vi "III_V_layer_v20.vi"(2 "Debug Mode":bool, 3 "Elapsed Time(s)":dbl, 4 "State":enum16{"Edit", "Start", "Run", "End", "Idle"}(ring), 5 "Argument List In":string[](array[string])) -> (0 "Status Out":string, 1 "Argument List Out":string[](array[string]))   [LabVIEW 2011]
uses:
  high_level_proc/Al_bubbler.ctl
  high_level_proc/In_bubbler.ctl
  high_level_proc/P_gas.ctl
  high_level_proc/As_gas.ctl
  high_level_proc/P_bubbler.ctl
  high_level_proc/bubblerDilution.ctl
panel:
  out "Zn bubbler Copy":T1={"Active"=FALSE, "main"={"Flow"=0.0, "Run"=FALSE, "Prep Ga"=FALSE, "Dilution"=FALSE, "Calculated"=0, "MFC2 flow"=10.0, "MFC3 flow"=100.0, "MFC1 flow"=0.0}} {"main"."MFC1 flow" format="%.4f"; "main"."MFC3 flow" format="%.1f"; "main"."MFC2 flow" format="%.2f"; "main"."Calculated" items=["Flow", "MFC1", "MFC2", "MFC3"]; "main"."Flow" format="%.2f"}
  in  "Zn bubbler":T1={"Active"=FALSE, "main"={"Flow"=0.0, "Run"=FALSE, "Prep Ga"=FALSE, "Dilution"=FALSE, "Calculated"=0, "MFC2 flow"=10.0, "MFC3 flow"=100.0, "MFC1 flow"=0.0}} {"main"."MFC1 flow" format="%.4f"; "main"."MFC3 flow" format="%.1f"; "main"."MFC2 flow" format="%.2f"; "main"."Calculated" items=["Flow", "MFC1", "MFC2", "MFC3"]; "main"."Flow" format="%.2f"}
  out "Se bubbler Copy":T1={"Active"=FALSE, "main"={"Flow"=0.0, "Run"=FALSE, "Prep Ga"=FALSE, "Dilution"=FALSE, "Calculated"=1, "MFC2 flow"=10.0, "MFC3 flow"=100.0, "MFC1 flow"=0.0}} {"main"."MFC1 flow" format="%.4f"; "main"."MFC3 flow" format="%.1f"; "main"."MFC2 flow" format="%.2f"; "main"."Calculated" items=["Ga flow", "MFC1", "MFC2", "MFC3"]; "main"."Flow" format="%.2f"}
  in  "Se bubbler":T1={"Active"=FALSE, "main"={"Flow"=0.0, "Run"=FALSE, "Prep Ga"=FALSE, "Dilution"=FALSE, "Calculated"=0, "MFC2 flow"=10.0, "MFC3 flow"=100.0, "MFC1 flow"=0.0}} {"main"."MFC1 flow" format="%.4f"; "main"."MFC3 flow" format="%.1f"; "main"."MFC2 flow" format="%.2f"; "main"."Calculated" items=["Flow", "MFC1", "MFC2", "MFC3"]; "main"."Flow" format="%.2f"}
  out "P bubbler Copy":T2 {"P bubbler main"."Flow" format="%.2f"}
  in  "P bubbler":T3 {"P bubbler main"."Flow" format="%.2f"}
  out "As gas Copy":T4 {"As gas main"."Flow" format="%.2f"}
  in  "As gas":T5 {"As gas main"."Flow" format="%.2f"}
  out "P gas Copy":T6 {"P gas main"."Flow" format="%.2f"}
  in  "P gas":T7 {"P gas main"."Flow" format="%.2f"}
  out "In bubbler Copy":T8 {"In main"."Flow" format="%.2f"}
  in  "In bubbler":T9 {"In main"."Flow" format="%.2f"}
  out "Ga bubbler Copy":T10={"Ga bubbler Active"=FALSE, "Ga main"={"Flow"=0.0, "Ga Run"=FALSE, "Prep Ga"=FALSE, "Dilution"=FALSE, "Ga Calculated"=1, "MFC2 flow"=10.0, "MFC3 flow"=100.0, "MFC1 flow"=0.0}} {"Ga main"."MFC1 flow" format="%.4f"; "Ga main"."MFC3 flow" format="%.1f"; "Ga main"."MFC2 flow" format="%.2f"; "Ga main"."Ga Calculated" items=["Ga flow", "MFC1", "MFC2", "MFC3"]; "Ga main"."Flow" format="%.2f"}
  in  "Ga bubbler":T1={"Active"=FALSE, "main"={"Flow"=0.0, "Run"=FALSE, "Prep Ga"=FALSE, "Dilution"=FALSE, "Calculated"=0, "MFC2 flow"=10.0, "MFC3 flow"=100.0, "MFC1 flow"=0.0}} {"main"."MFC1 flow" format="%.4f"; "main"."MFC3 flow" format="%.1f"; "main"."MFC2 flow" format="%.2f"; "main"."Calculated" items=["Flow", "MFC1", "MFC2", "MFC3"]; "main"."Flow" format="%.2f"}
  out "Al bubbler Copy":T11 {"Al main"."Al Flow" format="%.2f"}
  in  "Al bubbler":T12 {"Al main"."Al Flow" format="%.2f"}
  out "prep_done":bool
  out "run started":bool
  out "first":bool=TRUE
  out "total time":dbl
  out "is OK?":bool
  in  "prep_time":dbl
  in  "Cancel":bool
  in  "OK":bool
  out "tTotal(s) 2":dbl
  # "s"
  # "Add pre-run time to run time in editor."
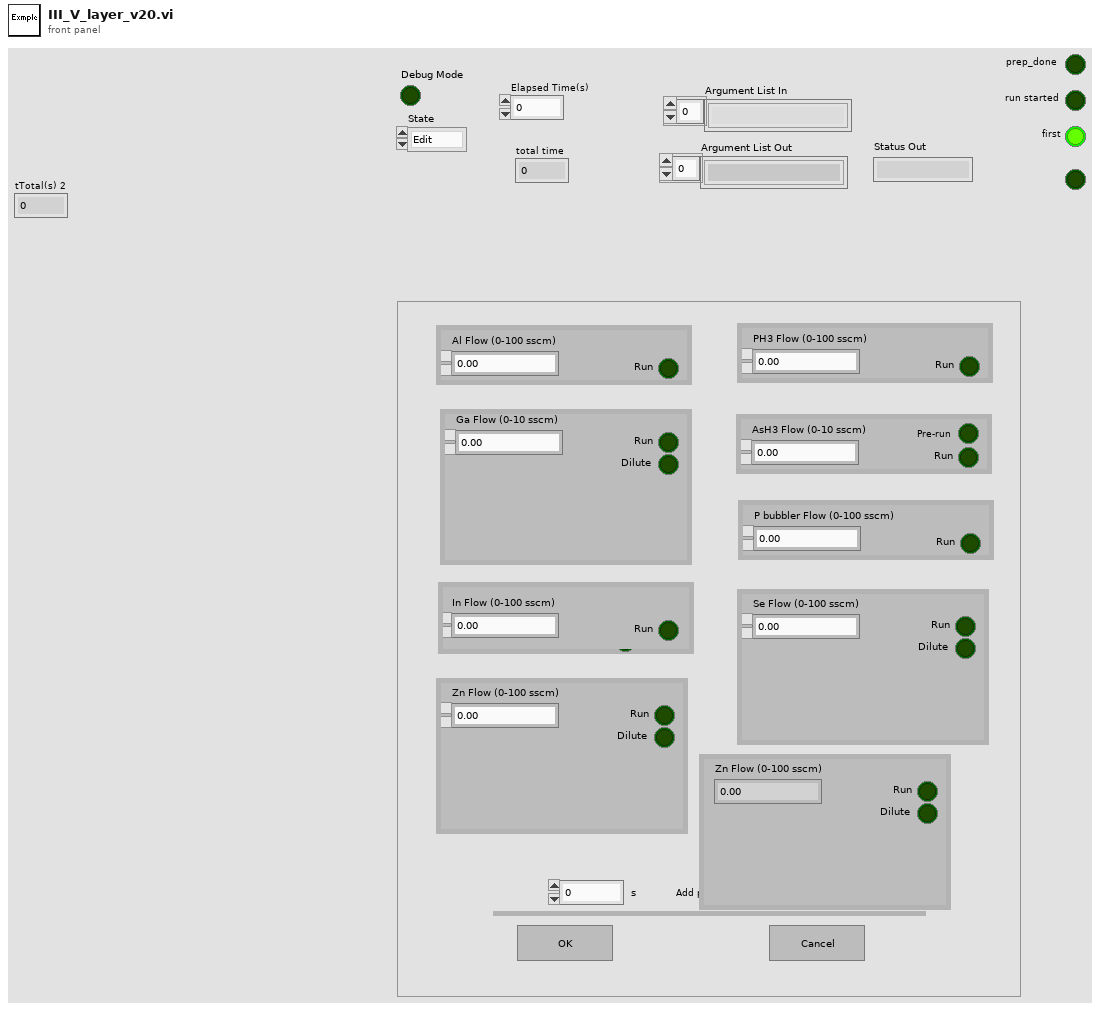
[diagram p1: front panel]
types:
  T1 = typedef "bubblerDilution.ctl" = cluster{"Active":bool, "main":cluster{"Flow":dbl, "Run":bool, "Prep Ga":bool, "Dilution":bool, "Calculated":u16, "MFC2 flow":dbl, "MFC3 flow":dbl, "MFC1 flow":dbl}}
  T2 = cluster{"P bubbler Active":bool, "P bubbler main":cluster{"Flow":dbl, "P bubbler Run":bool, "P bubbler Prep":bool}}
  T3 = typedef "P_bubbler.ctl" = cluster{"P bubbler Active":bool, "P bubbler main":cluster{"Flow":dbl, "P bubbler Run":bool, "P bubbler Prep":bool}}
  T4 = cluster{"As gas Active":bool, "As gas main":cluster{"Flow":dbl, "AsH3 Run":bool, "AsH3 Prep":bool}}
  T5 = typedef "As_gas.ctl" = cluster{"As gas Active":bool, "As gas main":cluster{"Flow":dbl, "AsH3 Run":bool, "AsH3 Prep":bool}}
  T6 = cluster{"P gas Active":bool, "P gas main":cluster{"Flow":dbl, "PH3 Run":bool, "PH3 Prep":bool}}
  T7 = typedef "P_gas.ctl" = cluster{"P gas Active":bool, "P gas main":cluster{"Flow":dbl, "PH3 Run":bool, "PH3 Prep":bool}}
  T8 = cluster{"In main":cluster{"Flow":dbl, "In Run":bool, "Prep In":bool}, "In bubbler Active":bool}
  T9 = typedef "In_bubbler.ctl" = cluster{"In main":cluster{"Flow":dbl, "In Run":bool, "Prep In":bool}, "In bubbler Active":bool}
  T10 = cluster{"Ga bubbler Active":bool, "Ga main":cluster{"Flow":dbl, "Ga Run":bool, "Prep Ga":bool, "Dilution":bool, "Ga Calculated":u16, "MFC2 flow":dbl, "MFC3 flow":dbl, "MFC1 flow":dbl}}
  T11 = cluster{"Al Active":bool, "Al main":cluster{"Al Flow":dbl, "Al Run":bool, "Prep Al":bool}}
  T12 = typedef "Al_bubbler.ctl" = cluster{"Al Active":bool, "Al main":cluster{"Al Flow":dbl, "Al Run":bool, "Prep Al":bool}}
  T13 = enum16{"Discrete", "Continuous", "Instantaneous", "Finite"}
  T14 = enum32{"Invalid", "Default", "Floating", "Floating/Auto-Hide", "Modal"}
  T15 = enum8{"Enabled", "Disabled", "Disabled and Grayed Out"}
  T16 = cluster{"Active":bool, "main":cluster{"Flow":dbl, "Run":bool, "Prep Ga":bool, "Dilution":bool, "Calculated":u16, "MFC2 flow":dbl, "MFC3 flow":dbl, "MFC1 flow":dbl}}
  T17 = cluster{"Al Flow":dbl, "Al Run":bool, "Prep Al":bool}
  T18 = cluster{"Flow":dbl, "Run":bool, "Prep Ga":bool, "Dilution":bool, "Calculated":u16, "MFC2 flow":dbl, "MFC3 flow":dbl, "MFC1 flow":dbl}
  T19 = cluster{"Flow":dbl, "In Run":bool, "Prep In":bool}
  T20 = cluster{"Flow":dbl, "PH3 Run":bool, "PH3 Prep":bool}
  T21 = cluster{"Flow":dbl, "AsH3 Run":bool, "AsH3 Prep":bool}
  T22 = cluster{"Flow":dbl, "P bubbler Run":bool, "P bubbler Prep":bool}
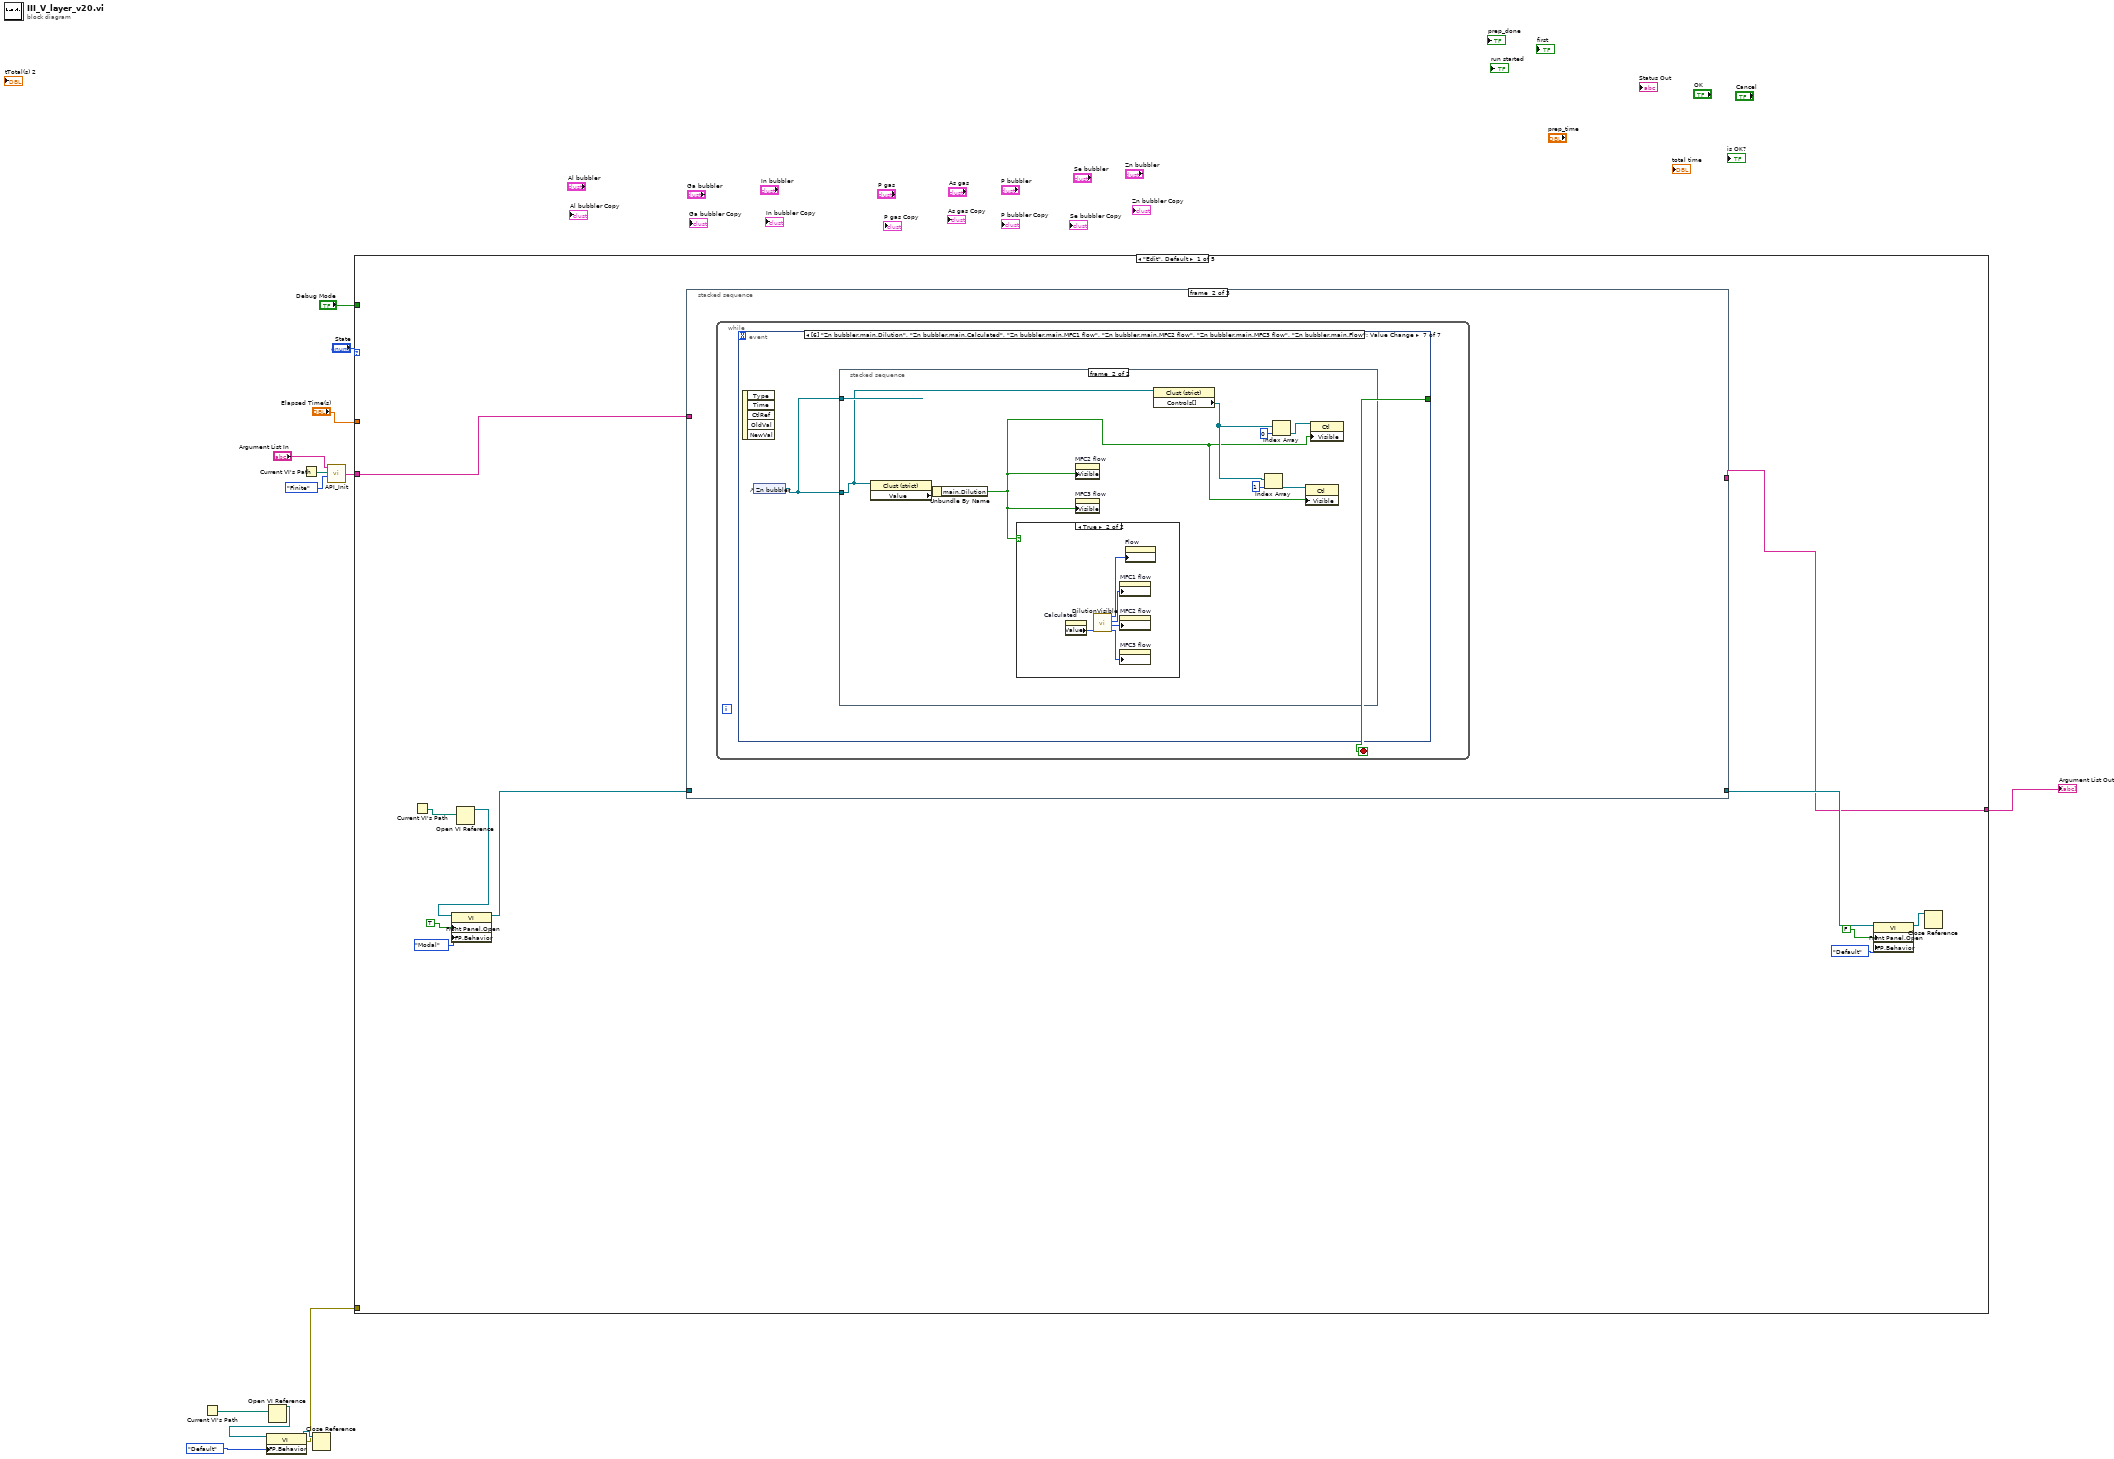
[diagram p0: block diagram]
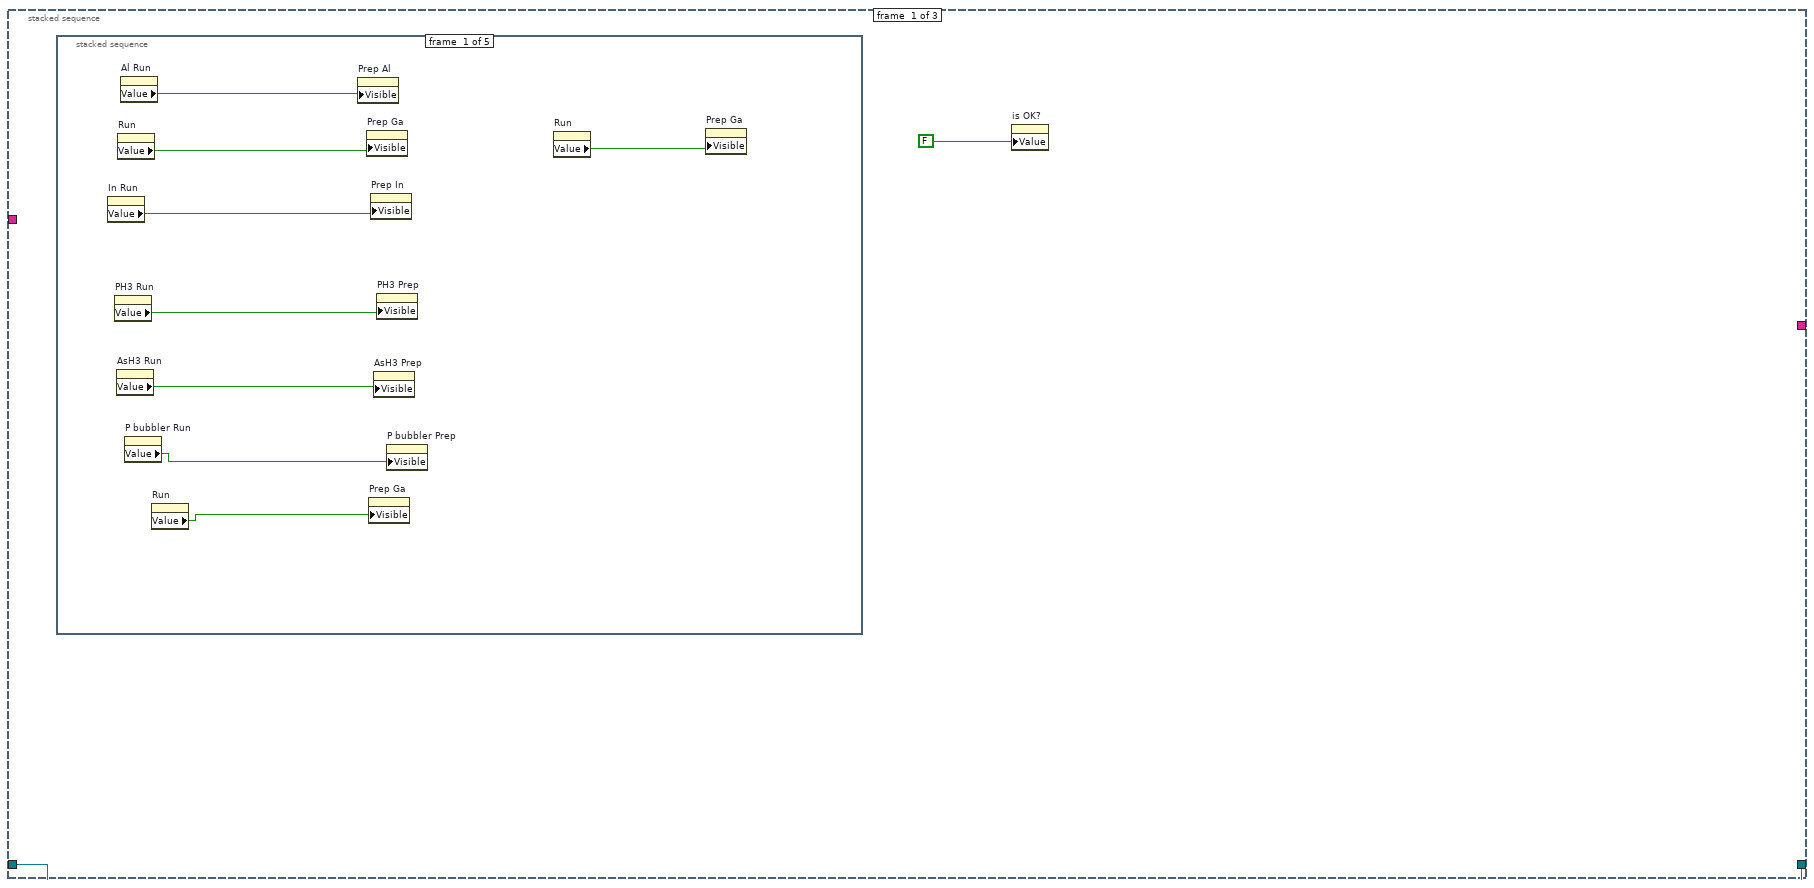
[diagram p2: hidden frame]
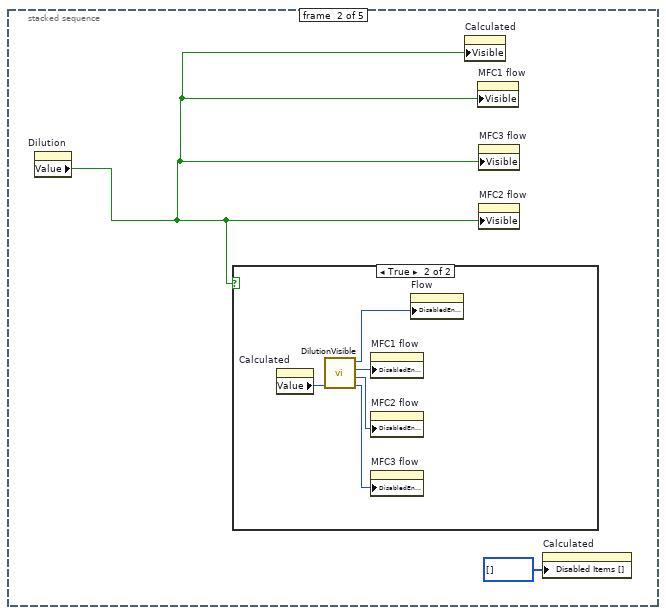
[diagram p3: hidden frame]
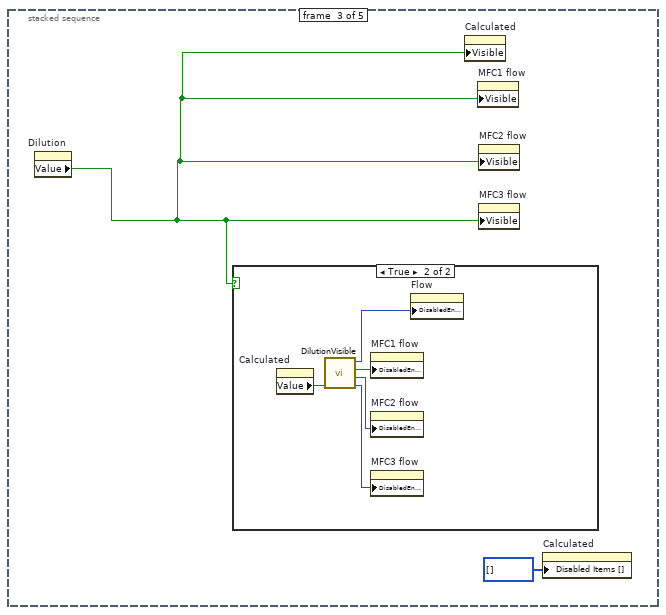
[diagram p5: hidden frame]
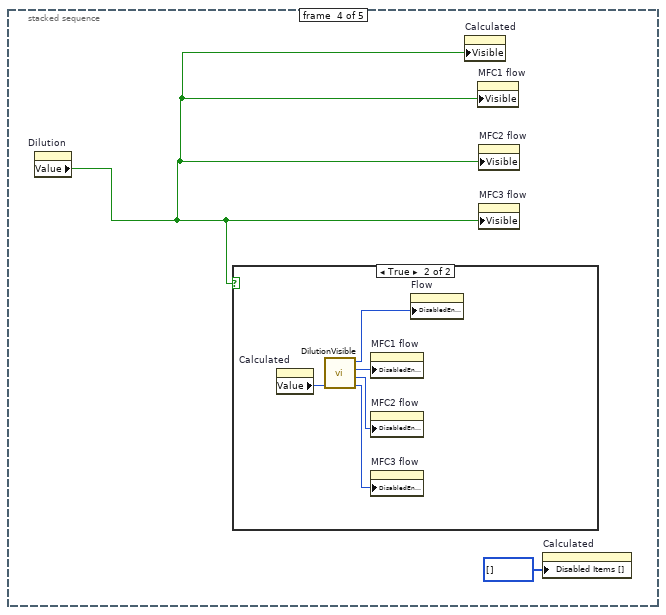
[diagram p7: hidden frame]
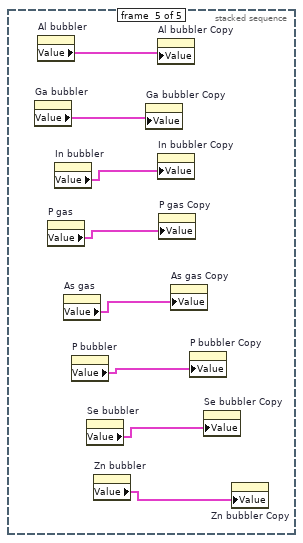
[diagram p9: hidden frame]
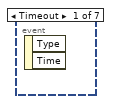
[diagram p10: hidden frame]
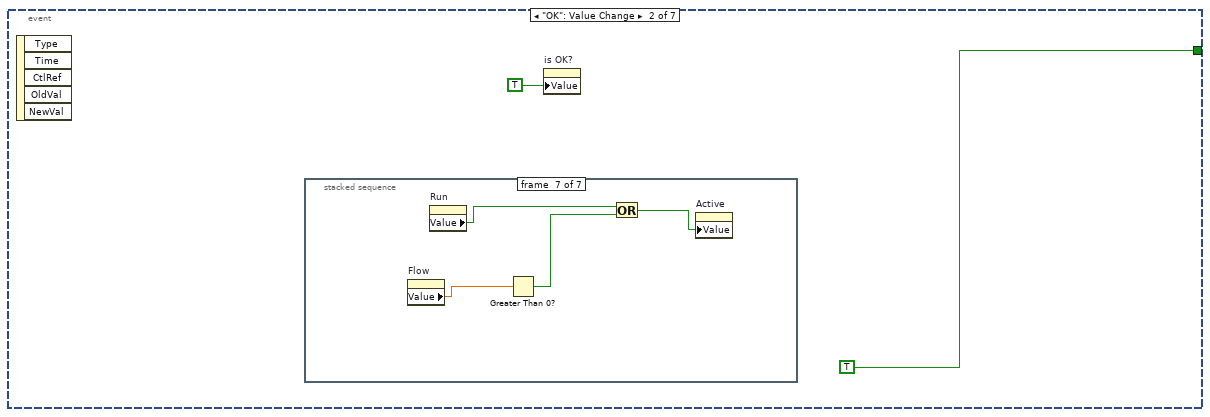
[diagram p11: hidden frame]
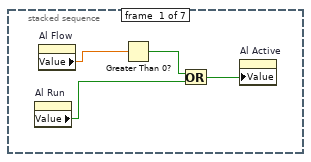
[diagram p12: hidden frame]
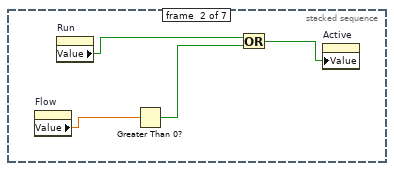
[diagram p13: hidden frame]
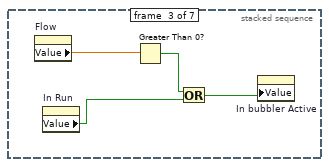
[diagram p14: hidden frame]
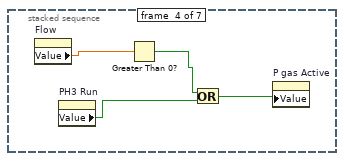
[diagram p15: hidden frame]
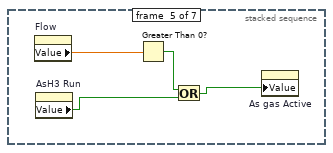
[diagram p16: hidden frame]
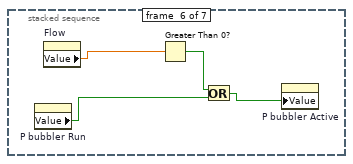
[diagram p17: hidden frame]
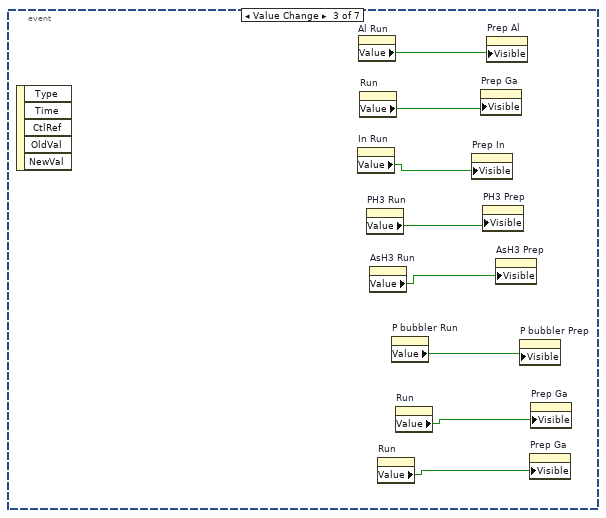
[diagram p18: hidden frame]
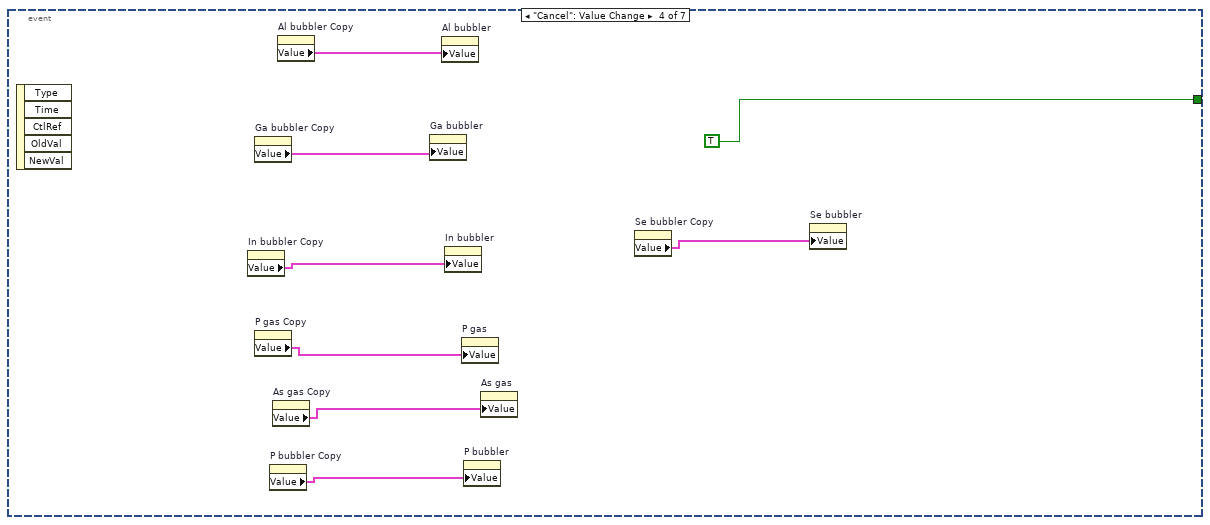
[diagram p19: hidden frame]
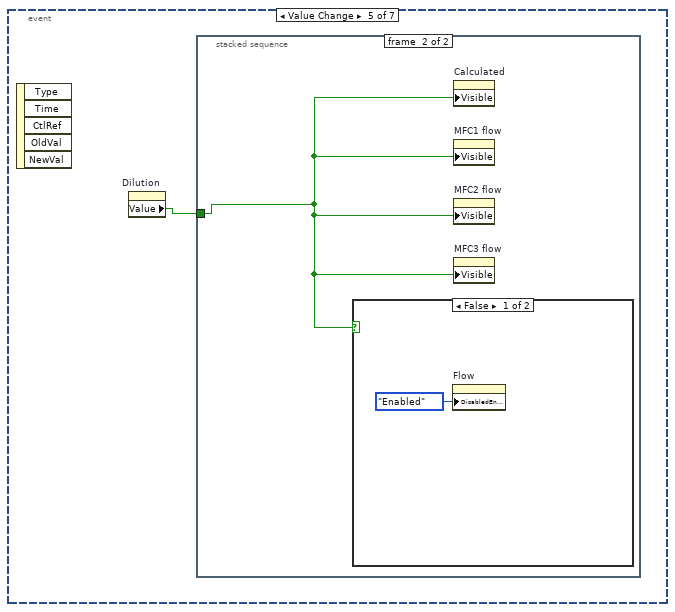
[diagram p20: hidden frame]
diagram:
  n1 = Current VI's Path() -> (path=w9:path)
  n2 = Open VI Reference(vi path=w9) -> (vi reference=w8:refnum<vi>)  [unwired: 1 in, 5 out]
  n3 = property class="VI"(reference=w8, "FP.Behavior"=T14."Default" ("Front Panel Window:Behavior")) -> (reference out=w6:refnum<vi>, error out=w5:errorcluster)  [unwired: 1 in]
  n4 = Current VI's Path() -> (path=w4:path)
  n5 = Close Reference(reference=w6) -> ()  [unwired: 1 in, 1 out]
  n6 = call "API_Init.vi"("API Mode"=T13."Finite", "VI Path"=w4, "Argument List In"="Argument List In") -> ("Argument List Out"=w1:string[])  [unwired: 1 in]
  n7 = case shown="\"Edit\", Default" "State" {
    tunnel: "Debug Mode" -> [_ w191 w208 _ _]
    tunnel: "Elapsed Time(s)" -> [_ _ w209 _ _]
    tunnel: w1 -> [w15 w195 w207 w318 w319]
    tunnel: [w14 w194 w206 w318 w319] -> w10
    tunnel: w5 -> [_ _ _ _ _]
    frame "Edit", Default {
      n8 = Current VI's Path() -> (path=w20:path)
      n9 = Open VI Reference(vi path=w20) -> (vi reference=w19:refnum<vi>)  [unwired: 1 in, 5 out]
      n10 = property class="VI"(reference=w19, "Front Panel.Open"=TRUE ("Front Panel Window:Open"), "FP.Behavior"=T14."Modal" ("Front Panel Window:Behavior")) -> (reference out=w18:refnum<vi>)  [unwired: 1 in, 1 out]
      n11 = stacked-sequence {
        tunnel: w15 -> [_ _ w186]
        tunnel: w18 -> [w26 _ _]
        tunnel: [w26 _ _] -> w22
        tunnel: [_ _ w187] -> w14
        frame #0 {
          n12 = stacked-sequence {
            frame #0 {
              n13 = property on="In Run" class="Bool (strict)"() -> ("Value"=w33:bool)  [unwired: 2 in, 2 out]
              n14 = property on="PH3 Run" class="Bool (strict)"() -> ("Value"=w31:bool)  [unwired: 2 in, 2 out]
              n15 = property on="AsH3 Run" class="Bool (strict)"() -> ("Value"=w30:bool)  [unwired: 2 in, 2 out]
              n16 = property on="Run" class="Bool (strict)"() -> ("Value"=w32:bool)  [unwired: 2 in, 2 out]
              n17 = property on="Al Run" class="Bool (strict)"() -> ("Value"=w34:bool)  [unwired: 2 in, 2 out]
              n18 = property on="P bubbler Run" class="Bool (strict)"() -> ("Value"=w29:bool)  [unwired: 2 in, 2 out]
              n19 = property on="Run" class="Bool (strict)"() -> ("Value"=w28:bool)  [unwired: 2 in, 2 out]
              n20 = property on="Prep Al" class="Bool (strict)"("Visible"=w34) -> ()  [unwired: 2 in, 2 out]
              n21 = property on="Prep Ga" class="Bool (strict)"("Visible"=w32) -> ()  [unwired: 2 in, 2 out]
              n22 = property on="Prep Ga" class="Bool (strict)"("Visible"=w28) -> ()  [unwired: 2 in, 2 out]
              n23 = property on="Prep In" class="Bool (strict)"("Visible"=w33) -> ()  [unwired: 2 in, 2 out]
              n24 = property on="AsH3 Prep" class="Bool (strict)"("Visible"=w30) -> ()  [unwired: 2 in, 2 out]
              n25 = property on="PH3 Prep" class="Bool (strict)"("Visible"=w31) -> ()  [unwired: 2 in, 2 out]
              n26 = property on="P bubbler Prep" class="Bool (strict)"("Visible"=w29) -> ()  [unwired: 2 in, 2 out]
              n27 = property on="Run" class="Bool (strict)"() -> ("Value"=w27:bool)  [unwired: 2 in, 2 out]
              n28 = property on="Prep Ga" class="Bool (strict)"("Visible"=w27) -> ()  [unwired: 2 in, 2 out]
            }
            frame #1 {
              n29 = property on="Dilution" class="Bool (strict)"() -> ("Value"=w36:bool)  [unwired: 2 in, 2 out]
              n30 = case shown="True" w36 {
                frame False {
                }
                frame True {
                  n31 = property on="Calculated" class="Ring (strict)"() -> ("Value"=w37:u16)  [unwired: 2 in, 2 out]
                  n32 = call "DilutionVisible.vi"("calculated"=w37) -> ("MFC3"=w40:u16, "MFC2"=w39:u16, "MFC1"=w38:u16, "flow"=w41:u16)  [unwired: 3 in]
                  n33 = property on="MFC1 flow" class="DigNum (strict)"("DisabledEnum"=w38) -> ()  [unwired: 2 in, 2 out]
                  n34 = property on="MFC2 flow" class="DigNum (strict)"("DisabledEnum"=w39) -> ()  [unwired: 2 in, 2 out]
                  n35 = property on="MFC3 flow" class="DigNum (strict)"("DisabledEnum"=w40) -> ()  [unwired: 2 in, 2 out]
                  n36 = property on="Flow" class="DigNum (strict)"("DisabledEnum"=w41) -> ()  [unwired: 2 in, 2 out]
                }
              }
              n37 = property on="Calculated" class="Ring (strict)"("Visible"=w36) -> ()  [unwired: 2 in, 2 out]
              n38 = property on="MFC1 flow" class="DigNum (strict)"("Visible"=w36) -> ()  [unwired: 2 in, 2 out]
              n39 = property on="MFC3 flow" class="DigNum (strict)"("Visible"=w36) -> ()  [unwired: 2 in, 2 out]
              n40 = property on="MFC2 flow" class="DigNum (strict)"("Visible"=w36) -> ()  [unwired: 2 in, 2 out]
              n41 = property on="Calculated" class="Ring (strict)"("Disabled Items []"=i32[] []) -> ()  [unwired: 2 in, 2 out]
            }
            frame #2 {
              n42 = property on="Dilution" class="Bool (strict)"() -> ("Value"=w43:bool)  [unwired: 2 in, 2 out]
              n43 = case shown="True" w43 {
                frame False {
                }
                frame True {
                  n44 = property on="Calculated" class="Ring (strict)"() -> ("Value"=w44:u16)  [unwired: 2 in, 2 out]
                  n45 = call "DilutionVisible.vi"("calculated"=w44) -> ("MFC3"=w47:u16, "MFC2"=w46:u16, "MFC1"=w45:u16, "flow"=w48:u16)  [unwired: 3 in]
                  n46 = property on="MFC1 flow" class="DigNum (strict)"("DisabledEnum"=w45) -> ()  [unwired: 2 in, 2 out]
                  n47 = property on="MFC2 flow" class="DigNum (strict)"("DisabledEnum"=w46) -> ()  [unwired: 2 in, 2 out]
                  n48 = property on="MFC3 flow" class="DigNum (strict)"("DisabledEnum"=w47) -> ()  [unwired: 2 in, 2 out]
                  n49 = property on="Flow" class="DigNum (strict)"("DisabledEnum"=w48) -> ()  [unwired: 2 in, 2 out]
                }
              }
              n50 = property on="Calculated" class="Ring (strict)"("Visible"=w43) -> ()  [unwired: 2 in, 2 out]
              n51 = property on="MFC1 flow" class="DigNum (strict)"("Visible"=w43) -> ()  [unwired: 2 in, 2 out]
              n52 = property on="MFC2 flow" class="DigNum (strict)"("Visible"=w43) -> ()  [unwired: 2 in, 2 out]
              n53 = property on="MFC3 flow" class="DigNum (strict)"("Visible"=w43) -> ()  [unwired: 2 in, 2 out]
              n54 = property on="Calculated" class="Ring (strict)"("Disabled Items []"=i32[] []) -> ()  [unwired: 2 in, 2 out]
            }
            frame #3 {
              n55 = property on="Dilution" class="Bool (strict)"() -> ("Value"=w50:bool)  [unwired: 2 in, 2 out]
              n56 = case shown="True" w50 {
                frame False {
                }
                frame True {
                  n57 = property on="Calculated" class="Ring (strict)"() -> ("Value"=w51:u16)  [unwired: 2 in, 2 out]
                  n58 = call "DilutionVisible.vi"("calculated"=w51) -> ("MFC3"=w54:u16, "MFC2"=w53:u16, "MFC1"=w52:u16, "flow"=w55:u16)  [unwired: 3 in]
                  n59 = property on="MFC1 flow" class="DigNum (strict)"("DisabledEnum"=w52) -> ()  [unwired: 2 in, 2 out]
                  n60 = property on="MFC2 flow" class="DigNum (strict)"("DisabledEnum"=w53) -> ()  [unwired: 2 in, 2 out]
                  n61 = property on="MFC3 flow" class="DigNum (strict)"("DisabledEnum"=w54) -> ()  [unwired: 2 in, 2 out]
                  n62 = property on="Flow" class="DigNum (strict)"("DisabledEnum"=w55) -> ()  [unwired: 2 in, 2 out]
                }
              }
              n63 = property on="Calculated" class="Ring (strict)"("Visible"=w50) -> ()  [unwired: 2 in, 2 out]
              n64 = property on="MFC1 flow" class="DigNum (strict)"("Visible"=w50) -> ()  [unwired: 2 in, 2 out]
              n65 = property on="MFC2 flow" class="DigNum (strict)"("Visible"=w50) -> ()  [unwired: 2 in, 2 out]
              n66 = property on="MFC3 flow" class="DigNum (strict)"("Visible"=w50) -> ()  [unwired: 2 in, 2 out]
              n67 = property on="Calculated" class="Ring (strict)"("Disabled Items []"=i32[] []) -> ()  [unwired: 2 in, 2 out]
            }
            frame #4 {
              n68 = property on="Ga bubbler" class="Clust (strict)"() -> ("Value"=w62:T16)  [unwired: 2 in, 2 out]
              n69 = property on="Al bubbler" class="Clust (strict)"() -> ("Value"=w63:T11)  [unwired: 2 in, 2 out]
              n70 = property on="P gas" class="Clust (strict)"() -> ("Value"=w60:T6)  [unwired: 2 in, 2 out]
              n71 = property on="In bubbler" class="Clust (strict)"() -> ("Value"=w61:T8)  [unwired: 2 in, 2 out]
              n72 = property on="As gas" class="Clust (strict)"() -> ("Value"=w59:T4)  [unwired: 2 in, 2 out]
              n73 = property on="P bubbler" class="Clust (strict)"() -> ("Value"=w58:T2)  [unwired: 2 in, 2 out]
              n74 = property on="Se bubbler" class="Clust (strict)"() -> ("Value"=w57:T16)  [unwired: 2 in, 2 out]
              n75 = property on="Zn bubbler" class="Clust (strict)"() -> ("Value"=w56:T16)  [unwired: 2 in, 2 out]
              n76 = property on="Ga bubbler Copy" class="Clust (strict)"("Value"=w62) -> ()  [unwired: 2 in, 2 out]
              n77 = property on="Al bubbler Copy" class="Clust (strict)"("Value"=w63) -> ()  [unwired: 2 in, 2 out]
              n78 = property on="In bubbler Copy" class="Clust (strict)"("Value"=w61) -> ()  [unwired: 2 in, 2 out]
              n79 = property on="P gas Copy" class="Clust (strict)"("Value"=w60) -> ()  [unwired: 2 in, 2 out]
              n80 = property on="As gas Copy" class="Clust (strict)"("Value"=w59) -> ()  [unwired: 2 in, 2 out]
              n81 = property on="P bubbler Copy" class="Clust (strict)"("Value"=w58) -> ()  [unwired: 2 in, 2 out]
              n82 = property on="Se bubbler Copy" class="Clust (strict)"("Value"=w57) -> ()  [unwired: 2 in, 2 out]
              n83 = property on="Zn bubbler Copy" class="Clust (strict)"("Value"=w56) -> ()  [unwired: 2 in, 2 out]
            }
          }
          n84 = property on="is OK?" class="Bool (strict)"("Value"=FALSE ("is OK?")) -> ()  [unwired: 2 in, 2 out]
        }
        frame #1 {
          n85 = while {
            stop <- w64 stop-if-true
            n86 = event shown="[6] \"Zn bubbler.main.Dilution\", \"Zn bubbler.main.Calculated\", \"Zn bubbler.main.MFC1 flow\", \"Zn bubbler.main.MFC2 flow\", \"Zn bubbler.main.MFC3 flow\", \"Zn bubbler.main.Flow\": Value Change" {
              selector: _ -> [_ _ _ _ _ _ _]
              dyn-events: _ -> [_ _ _ _ _ _ _]
              timeout: _ -> [_ _ _ _ _ _ _]
              tunnel: [_ TRUE _ TRUE _ _ _] -> w64
              event Timeout {
                n87 = event-data() -> ()  [unwired: 1 in, 2 out]
              }
              event "OK": Value Change {
                n88 = event-data() -> ()  [unwired: 1 in, 5 out]
                n89 = stacked-sequence {
                  frame #0 {
                    n90 = property on="Al Run" class="Bool (strict)"() -> ("Value"=w68:bool)  [unwired: 2 in, 2 out]
                    n91 = property on="Al Flow" class="DigNum (strict)"() -> ("Value"=w69:dbl)  [unwired: 2 in, 2 out]
                    n92 = Greater Than 0?(x=w69) -> (x > 0?=w70:bool)
                    n93 = Or(x=w70, y=w68) -> (x .or. y?=w67:bool)
                    n94 = property on="Al Active" class="Bool (strict)"("Value"=w67) -> ()  [unwired: 2 in, 2 out]
                  }
                  frame #1 {
                    n95 = property on="Flow" class="DigNum (strict)"() -> ("Value"=w71:dbl)  [unwired: 2 in, 2 out]
                    n96 = property on="Run" class="Bool (strict)"() -> ("Value"=w72:bool)  [unwired: 2 in, 2 out]
                    n97 = Greater Than 0?(x=w71) -> (x > 0?=w74:bool)
                    n98 = Or(x=w72, y=w74) -> (x .or. y?=w73:bool)
                    n99 = property on="Active" class="Bool (strict)"("Value"=w73) -> ()  [unwired: 2 in, 2 out]
                  }
                  frame #2 {
                    n100 = property on="Flow" class="DigNum (strict)"() -> ("Value"=w77:dbl)  [unwired: 2 in, 2 out]
                    n101 = property on="In Run" class="Bool (strict)"() -> ("Value"=w76:bool)  [unwired: 2 in, 2 out]
                    n102 = Greater Than 0?(x=w77) -> (x > 0?=w78:bool)
                    n103 = Or(x=w78, y=w76) -> (x .or. y?=w75:bool)
                    n104 = property on="In bubbler Active" class="Bool (strict)"("Value"=w75) -> ()  [unwired: 2 in, 2 out]
                  }
                  frame #3 {
                    n105 = property on="Flow" class="DigNum (strict)"() -> ("Value"=w81:dbl)  [unwired: 2 in, 2 out]
                    n106 = property on="PH3 Run" class="Bool (strict)"() -> ("Value"=w80:bool)  [unwired: 2 in, 2 out]
                    n107 = Greater Than 0?(x=w81) -> (x > 0?=w82:bool)
                    n108 = Or(x=w82, y=w80) -> (x .or. y?=w79:bool)
                    n109 = property on="P gas Active" class="Bool (strict)"("Value"=w79) -> ()  [unwired: 2 in, 2 out]
                  }
                  frame #4 {
                    n110 = property on="Flow" class="DigNum (strict)"() -> ("Value"=w85:dbl)  [unwired: 2 in, 2 out]
                    n111 = property on="AsH3 Run" class="Bool (strict)"() -> ("Value"=w84:bool)  [unwired: 2 in, 2 out]
                    n112 = Greater Than 0?(x=w85) -> (x > 0?=w86:bool)
                    n113 = Or(x=w86, y=w84) -> (x .or. y?=w83:bool)
                    n114 = property on="As gas Active" class="Bool (strict)"("Value"=w83) -> ()  [unwired: 2 in, 2 out]
                  }
                  frame #5 {
                    n115 = property on="P bubbler Run" class="Bool (strict)"() -> ("Value"=w88:bool)  [unwired: 2 in, 2 out]
                    n116 = property on="Flow" class="DigNum (strict)"() -> ("Value"=w89:dbl)  [unwired: 2 in, 2 out]
                    n117 = Greater Than 0?(x=w89) -> (x > 0?=w90:bool)
                    n118 = Or(x=w90, y=w88) -> (x .or. y?=w87:bool)
                    n119 = property on="P bubbler Active" class="Bool (strict)"("Value"=w87) -> ()  [unwired: 2 in, 2 out]
                  }
                  frame #6 {
                    n120 = property on="Flow" class="DigNum (strict)"() -> ("Value"=w91:dbl)  [unwired: 2 in, 2 out]
                    n121 = property on="Run" class="Bool (strict)"() -> ("Value"=w92:bool)  [unwired: 2 in, 2 out]
                    n122 = Greater Than 0?(x=w91) -> (x > 0?=w94:bool)
                    n123 = Or(x=w92, y=w94) -> (x .or. y?=w93:bool)
                    n124 = property on="Active" class="Bool (strict)"("Value"=w93) -> ()  [unwired: 2 in, 2 out]
                  }
                }
                n125 = property on="is OK?" class="Bool (strict)"("Value"=TRUE ("is OK?")) -> ()  [unwired: 2 in, 2 out]
              }
              event Value Change {
                n126 = event-data() -> ()  [unwired: 1 in, 5 out]
                n127 = property on="In Run" class="Bool (strict)"() -> ("Value"=w99:bool)  [unwired: 2 in, 2 out]
                n128 = property on="Al Run" class="Bool (strict)"() -> ("Value"=w101:bool)  [unwired: 2 in, 2 out]
                n129 = property on="Run" class="Bool (strict)"() -> ("Value"=w100:bool)  [unwired: 2 in, 2 out]
                n130 = property on="PH3 Run" class="Bool (strict)"() -> ("Value"=w98:bool)  [unwired: 2 in, 2 out]
                n131 = property on="AsH3 Run" class="Bool (strict)"() -> ("Value"=w97:bool)  [unwired: 2 in, 2 out]
                n132 = property on="Run" class="Bool (strict)"() -> ("Value"=w95:bool)  [unwired: 2 in, 2 out]
                n133 = property on="P bubbler Run" class="Bool (strict)"() -> ("Value"=w102:bool)  [unwired: 2 in, 2 out]
                n134 = property on="Run" class="Bool (strict)"() -> ("Value"=w96:bool)  [unwired: 2 in, 2 out]
                n135 = property on="Prep In" class="Bool (strict)"("Visible"=w99) -> ()  [unwired: 2 in, 2 out]
                n136 = property on="Prep Ga" class="Bool (strict)"("Visible"=w100) -> ()  [unwired: 2 in, 2 out]
                n137 = property on="PH3 Prep" class="Bool (strict)"("Visible"=w98) -> ()  [unwired: 2 in, 2 out]
                n138 = property on="Prep Al" class="Bool (strict)"("Visible"=w101) -> ()  [unwired: 2 in, 2 out]
                n139 = property on="AsH3 Prep" class="Bool (strict)"("Visible"=w97) -> ()  [unwired: 2 in, 2 out]
                n140 = property on="P bubbler Prep" class="Bool (strict)"("Visible"=w102) -> ()  [unwired: 2 in, 2 out]
                n141 = property on="Prep Ga" class="Bool (strict)"("Visible"=w95) -> ()  [unwired: 2 in, 2 out]
                n142 = property on="Prep Ga" class="Bool (strict)"("Visible"=w96) -> ()  [unwired: 2 in, 2 out]
              }
              event "Cancel": Value Change {
                n143 = event-data() -> ()  [unwired: 1 in, 5 out]
                n144 = property on="In bubbler Copy" class="Clust (strict)"() -> ("Value"=w108:T8)  [unwired: 2 in, 2 out]
                n145 = property on="Ga bubbler Copy" class="Clust (strict)"() -> ("Value"=w107:T10)  [unwired: 2 in, 2 out]
                n146 = property on="P gas Copy" class="Clust (strict)"() -> ("Value"=w106:T6)  [unwired: 2 in, 2 out]
                n147 = property on="P bubbler Copy" class="Clust (strict)"() -> ("Value"=w104:T2)  [unwired: 2 in, 2 out]
                n148 = property on="As gas Copy" class="Clust (strict)"() -> ("Value"=w105:T4)  [unwired: 2 in, 2 out]
                n149 = property on="Al bubbler Copy" class="Clust (strict)"() -> ("Value"=w109:T11)  [unwired: 2 in, 2 out]
                n150 = property on="Ga bubbler" class="Clust (strict)"("Value"=w107) -> ()  [unwired: 2 in, 2 out]
                n151 = property on="Al bubbler" class="Clust (strict)"("Value"=w109) -> ()  [unwired: 2 in, 2 out]
                n152 = property on="In bubbler" class="Clust (strict)"("Value"=w108) -> ()  [unwired: 2 in, 2 out]
                n153 = property on="P gas" class="Clust (strict)"("Value"=w106) -> ()  [unwired: 2 in, 2 out]
                n154 = property on="P bubbler" class="Clust (strict)"("Value"=w104) -> ()  [unwired: 2 in, 2 out]
                n155 = property on="As gas" class="Clust (strict)"("Value"=w105) -> ()  [unwired: 2 in, 2 out]
                n156 = property on="Se bubbler Copy" class="Clust (strict)"() -> ("Value"=w103:T16)  [unwired: 2 in, 2 out]
                n157 = property on="Se bubbler" class="Clust (strict)"("Value"=w103) -> ()  [unwired: 2 in, 2 out]
              }
              event Value Change {
                n158 = event-data() -> ()  [unwired: 1 in, 5 out]
                n159 = property on="Dilution" class="Bool (strict)"() -> ("Value"=w111:bool)  [unwired: 2 in, 2 out]
                n160 = stacked-sequence {
                  tunnel: w111 -> [w112 w122]
                  frame #0 {
                    n161 = case shown="True" w112 {
                      frame False {
                      }
                      frame True {
                        n162 = property on="Flow" class="DigNum (strict)"() -> ("Value"=w120:dbl)  [unwired: 2 in, 2 out]
                        n163 = property on="Calculated" class="Ring (strict)"() -> ("Value"=w121:u16)  [unwired: 2 in, 2 out]
                        n164 = property on="MFC1 flow" class="DigNum (strict)"() -> ("Value"=w119:dbl)  [unwired: 2 in, 2 out]
                        n165 = property on="MFC2 flow" class="DigNum (strict)"() -> ("Value"=w118:dbl)  [unwired: 2 in, 2 out]
                        n166 = property on="MFC3 flow" class="DigNum (strict)"() -> ("Value"=w117:dbl)  [unwired: 2 in, 2 out]
                        n167 = call "dilutionCalc.vi"("Calculated"=w121, "MFC3"=w117, "MFC2"=w118, "MFC1"=w119, "flow"=w120) -> ("MFC3 out"=w113:dbl, "MFC2 out"=w114:dbl, "MFC1 out"=w115:dbl, "flow out"=w116:dbl)  [unwired: 1 in]
                        n168 = property on="MFC1 flow" class="DigNum (strict)"("Value"=w115) -> ()  [unwired: 2 in, 2 out]
                        n169 = property on="Flow" class="DigNum (strict)"("Value"=w116) -> ()  [unwired: 2 in, 2 out]
                        n170 = property on="MFC3 flow" class="DigNum (strict)"("Value"=w113) -> ()  [unwired: 2 in, 2 out]
                        n171 = property on="MFC2 flow" class="DigNum (strict)"("Value"=w114) -> ()  [unwired: 2 in, 2 out]
                      }
                    }
                  }
                  frame #1 {
                    n172 = case shown="False" w122 {
                      frame False {
                        n173 = property on="Flow" class="DigNum (strict)"("DisabledEnum"=T15."Enabled" ("Disabled")) -> ()  [unwired: 2 in, 2 out]
                      }
                      frame True {
                        n174 = property on="Calculated" class="Ring (strict)"() -> ("Value"=w124:u16)  [unwired: 2 in, 2 out]
                        n175 = call "DilutionVisible.vi"("calculated"=w124) -> ("MFC3"=w128:u16, "MFC2"=w127:u16, "MFC1"=w126:u16, "flow"=w125:u16)  [unwired: 3 in]
                        n176 = property on="MFC1 flow" class="DigNum (strict)"("DisabledEnum"=w126) -> ()  [unwired: 2 in, 2 out]
                        n177 = property on="MFC2 flow" class="DigNum (strict)"("DisabledEnum"=w127) -> ()  [unwired: 2 in, 2 out]
                        n178 = property on="MFC3 flow" class="DigNum (strict)"("DisabledEnum"=w128) -> ()  [unwired: 2 in, 2 out]
                        n179 = property on="Flow" class="DigNum (strict)"("DisabledEnum"=w125) -> ()  [unwired: 2 in, 2 out]
                      }
                    }
                    n180 = property on="Calculated" class="Ring (strict)"("Visible"=w122) -> ()  [unwired: 2 in, 2 out]
                    n181 = property on="MFC1 flow" class="DigNum (strict)"("Visible"=w122) -> ()  [unwired: 2 in, 2 out]
                    n182 = property on="MFC2 flow" class="DigNum (strict)"("Visible"=w122) -> ()  [unwired: 2 in, 2 out]
                    n183 = property on="MFC3 flow" class="DigNum (strict)"("Visible"=w122) -> ()  [unwired: 2 in, 2 out]
                  }
                }
              }
              event Value Change {
                n184 = event-data() -> ()  [unwired: 1 in, 5 out]
                n185 = property on="Dilution" class="Bool (strict)"() -> ("Value"=w129:bool)  [unwired: 2 in, 2 out]
                n186 = stacked-sequence {
                  tunnel: w129 -> [w130 w140]
                  frame #0 {
                    n187 = case shown="True" w130 {
                      frame False {
                      }
                      frame True {
                        n188 = property on="Flow" class="DigNum (strict)"() -> ("Value"=w138:dbl)  [unwired: 2 in, 2 out]
                        n189 = property on="Calculated" class="Ring (strict)"() -> ("Value"=w139:u16)  [unwired: 2 in, 2 out]
                        n190 = property on="MFC1 flow" class="DigNum (strict)"() -> ("Value"=w137:dbl)  [unwired: 2 in, 2 out]
                        n191 = property on="MFC2 flow" class="DigNum (strict)"() -> ("Value"=w136:dbl)  [unwired: 2 in, 2 out]
                        n192 = property on="MFC3 flow" class="DigNum (strict)"() -> ("Value"=w135:dbl)  [unwired: 2 in, 2 out]
                        n193 = call "dilutionCalc.vi"("Calculated"=w139, "MFC3"=w135, "MFC2"=w136, "MFC1"=w137, "flow"=w138) -> ("MFC3 out"=w131:dbl, "MFC2 out"=w132:dbl, "MFC1 out"=w133:dbl, "flow out"=w134:dbl)  [unwired: 1 in]
                        n194 = property on="MFC1 flow" class="DigNum (strict)"("Value"=w133) -> ()  [unwired: 2 in, 2 out]
                        n195 = property on="Flow" class="DigNum (strict)"("Value"=w134) -> ()  [unwired: 2 in, 2 out]
                        n196 = property on="MFC3 flow" class="DigNum (strict)"("Value"=w131) -> ()  [unwired: 2 in, 2 out]
                        n197 = property on="MFC2 flow" class="DigNum (strict)"("Value"=w132) -> ()  [unwired: 2 in, 2 out]
                      }
                    }
                  }
                  frame #1 {
                    n198 = case shown="True" w140 {
                      frame False {
                        n199 = property on="Flow" class="DigNum (strict)"("DisabledEnum"=T15."Enabled" ("Disabled")) -> ()  [unwired: 2 in, 2 out]
                      }
                      frame True {
                        n200 = property on="Calculated" class="Ring (strict)"() -> ("Value"=w142:u16)  [unwired: 2 in, 2 out]
                        n201 = call "DilutionVisible.vi"("calculated"=w142) -> ("MFC3"=w146:u16, "MFC2"=w145:u16, "MFC1"=w144:u16, "flow"=w143:u16)  [unwired: 3 in]
                        n202 = property on="MFC1 flow" class="DigNum (strict)"("DisabledEnum"=w144) -> ()  [unwired: 2 in, 2 out]
                        n203 = property on="MFC2 flow" class="DigNum (strict)"("DisabledEnum"=w145) -> ()  [unwired: 2 in, 2 out]
                        n204 = property on="MFC3 flow" class="DigNum (strict)"("DisabledEnum"=w146) -> ()  [unwired: 2 in, 2 out]
                        n205 = property on="Flow" class="DigNum (strict)"("DisabledEnum"=w143) -> ()  [unwired: 2 in, 2 out]
                      }
                    }
                    n206 = property on="Calculated" class="Ring (strict)"("Visible"=w140) -> ()  [unwired: 2 in, 2 out]
                    n207 = property on="MFC1 flow" class="DigNum (strict)"("Visible"=w140) -> ()  [unwired: 2 in, 2 out]
                    n208 = property on="MFC2 flow" class="DigNum (strict)"("Visible"=w140) -> ()  [unwired: 2 in, 2 out]
                    n209 = property on="MFC3 flow" class="DigNum (strict)"("Visible"=w140) -> ()  [unwired: 2 in, 2 out]
                  }
                }
              }
              event Value Change {
                n210 = event-data() -> ()  [unwired: 1 in, 5 out]
                n211 = control-ref of="Zn bubbler"() -> (w147:refnum<vi>)
                n212 = stacked-sequence {
                  tunnel: w147 -> [w156 _]
                  tunnel: w147 -> [w155 w177]
                  frame #0 {
                    n213 = property class="Clust (strict)"(reference=w155) -> ("Value"=w154:T16)  [unwired: 1 in, 2 out]
                    n214 = Unbundle By Name(w154) -> ("main.Dilution"=w152:bool, "main.Calculated"=w153:u16, "main.Flow"=w151:dbl, "main.MFC1 flow"=w150:dbl, "main.MFC2 flow"=w149:dbl, "main.MFC3 flow"=w148:dbl)
                    n215 = case shown="True" w152 {
                      tunnel: w153 -> [_ w170]
                      tunnel: w151 -> [_ w169]
                      tunnel: w150 -> [_ w168]
                      tunnel: w149 -> [_ w167]
                      tunnel: w148 -> [_ w166]
                      tunnel: [_ w165] -> w161
                      tunnel: [_ w164] -> w160
                      tunnel: [_ w163] -> w159
                      tunnel: [_ w162] -> w158
                      frame False {
                      }
                      frame True {
                        n216 = call "dilutionCalc.vi"("Calculated"=w170, "MFC3"=w166, "MFC2"=w167, "MFC1"=w168, "flow"=w169) -> ("MFC3 out"=w162:dbl, "MFC2 out"=w163:dbl, "MFC1 out"=w164:dbl, "flow out"=w165:dbl)  [unwired: 1 in]
                      }
                    }
                    n217 = Bundle By Name(cluster=w154, "main.Flow"=w161, "main.MFC1 flow"=w160, "main.MFC2 flow"=w159, "main.MFC3 flow"=w158) -> (w157:T16)
                    n218 = property class="Clust (strict)"(reference=w156, "Value"=w157) -> ()  [unwired: 1 in, 2 out]
                  }
                  frame #1 {
                    n219 = property class="Clust (strict)"(reference=w177) -> ("Value"=w178:T16)  [unwired: 1 in, 2 out]
                    n220 = Unbundle By Name(w178) -> ("main.Dilution"=w171:bool)
                    n221 = case shown="True" w171 {
                      frame False {
                        n222 = property on="Flow" class="DigNum (strict)"("DisabledEnum"=T15."Enabled" ("Disabled")) -> ()  [unwired: 2 in, 2 out]
                      }
                      frame True {
                        n223 = property on="Calculated" class="Ring (strict)"() -> ("Value"=w180:u16)  [unwired: 2 in, 2 out]
                        n224 = call "DilutionVisible.vi"("calculated"=w180) -> ("MFC3"=w184:u16, "MFC2"=w183:u16, "MFC1"=w182:u16, "flow"=w181:u16)  [unwired: 3 in]
                        n225 = property on="MFC1 flow" class="DigNum (strict)"("DisabledEnum"=w182) -> ()  [unwired: 2 in, 2 out]
                        n226 = property on="MFC2 flow" class="DigNum (strict)"("DisabledEnum"=w183) -> ()  [unwired: 2 in, 2 out]
                        n227 = property on="MFC3 flow" class="DigNum (strict)"("DisabledEnum"=w184) -> ()  [unwired: 2 in, 2 out]
                        n228 = property on="Flow" class="DigNum (strict)"("DisabledEnum"=w181) -> ()  [unwired: 2 in, 2 out]
                      }
                    }
                    n229 = property on="MFC2 flow" class="DigNum (strict)"("Visible"=w171) -> ()  [unwired: 2 in, 2 out]
                    n230 = property on="MFC3 flow" class="DigNum (strict)"("Visible"=w171) -> ()  [unwired: 2 in, 2 out]
                    n231 = property class="Clust (strict)"(reference=w177) -> ("Controls[]"=w173:refnum<vi>[])  [unwired: 1 in, 2 out]
                    n232 = Index Array(array=w173, index=1) -> (element=w172:refnum<vi>)
                    n233 = Index Array(array=w173, index=0) -> (element=w175:refnum<vi>)
                    n234 = property class="Ctl"(reference=w172, "Visible"=w171) -> ()  [unwired: 1 in, 2 out]
                    n235 = property class="Ctl"(reference=w175, "Visible"=w171) -> ()  [unwired: 1 in, 2 out]
                  }
                }
              }
            }
          }
        }
        frame #2 {
          n236 = property on="is OK?" class="Bool (strict)"() -> ("Value"=w185:bool)  [unwired: 2 in, 2 out]
          n237 = Not(x=w185) -> (.not. x?=w189:bool)
          n238 = Current VI's Path() -> (path=w188:path)
          n239 = call "API_Edit.vi"("Cancel"=w189, "OK"=w185, "VI Path"=w188, "Argument List In"=w186) -> ("Argument List Out"=w187:string[])
        }
      }
      n240 = property class="VI"(reference=w22, "Front Panel.Open"=FALSE ("Front Panel Window:Open"), "FP.Behavior"=T14."Default" ("Front Panel Window:Behavior")) -> (reference out=w23:refnum<vi>)  [unwired: 1 in, 1 out]
      n241 = Close Reference(reference=w23) -> ()  [unwired: 1 in, 1 out]
    }
    frame "Start" {
      n242 = call "Set_Argument.vi"("Enable"=FALSE, "Argument"="run_started", "Argument List In"=w195) -> ("Argument List Out"=w194:string[])
      n243 = property on="prep_time" class="DigNum (strict)"() -> ("Value"=w193:dbl)  [unwired: 2 in, 2 out]
      n244 = Greater Than 0?(x=w193) -> (x > 0?=w192:bool)
      n245 = And(x=w191, y=w192) -> (x .and. y?=w190:bool)
      n246 = case shown="False" w190 {
        frame False {
          n247 = property on="In bubbler" class="Clust (strict)"() -> ("Value"=w203:T8)  [unwired: 2 in, 2 out]
          n248 = property on="Ga bubbler" class="Clust (strict)"() -> ("Value"=w204:T16)  [unwired: 2 in, 2 out]
          n249 = property on="Al bubbler" class="Clust (strict)"() -> ("Value"=w205:T11)  [unwired: 2 in, 2 out]
          n250 = property on="Se bubbler" class="Clust (strict)"() -> ("Value"=w198:T16)  [unwired: 2 in, 2 out]
          n251 = property on="P bubbler" class="Clust (strict)"() -> ("Value"=w200:T2)  [unwired: 2 in, 2 out]
          n252 = property on="P gas" class="Clust (strict)"() -> ("Value"=w202:T6)  [unwired: 2 in, 2 out]
          n253 = property on="As gas" class="Clust (strict)"() -> ("Value"=w201:T4)  [unwired: 2 in, 2 out]
          n254 = call "Set_V_III.vi"("Se bubbler"=w198, "P bubbler"=w200, "As gas"=w201, "P gas"=w202, "Run Started"=FALSE, "In bubbler"=w203, "Ga bubbler"=w204, "Al bubbler"=w205) -> ()  [unwired: 4 in]
        }
        frame True {
        }
      }
    }
    frame "Run" {
      n255 = stacked-sequence {
        tunnel: w209 -> [_ w214 _ _]
        tunnel: w207 -> [w211 _ _ w295]
        tunnel: w208 -> [_ _ _ w293]
        tunnel: [_ _ _ w294] -> w206
        frame #0 {
          n256 = call "Get_Argument.vi"("Argument"="run_started", "Argument List"=w211) -> ("Enabled"=w210:bool)
          n257 = local write "run started"(w210) -> ()
        }
        frame #1 {
          n258 = property on="prep_time" class="DigNum (strict)"() -> ("Value"=w215:dbl)  [unwired: 2 in, 2 out]
          n259 = Greater Or Equal?(x=w214, y=w215) -> (x >= y?=w213:bool)
          n260 = local write "prep_done"(w213) -> ()
        }
        frame #2 {
          n261 = local read "run started"() -> (w217:bool)
          n262 = Not(x=w217) -> (.not. x?=w216:bool)
          n263 = stacked-sequence {
            tunnel: w216 -> [w219 w226 w236 w246 w256 w266 w276 w286]
            frame #0 {
              n264 = case shown="False" w219 {
                tunnel: ["run: " "pre-run: "] -> w218
                frame False {
                }
                frame True {
                }
              }
              n265 = property on="Status Out" class="Str"("Value"=w218) -> ()  [unwired: 2 in, 2 out]
            }
            frame #1 {
              n266 = property on="Al main" class="Clust (strict)"() -> ("Value"=w224:T17)  [unwired: 2 in, 2 out]
              n267 = property on="Al Active" class="Bool (strict)"() -> ("Value"=w225:bool)  [unwired: 2 in, 2 out]
              n268 = property on="Status Out" class="Str"() -> ("Value"=w231:string)  [unwired: 2 in, 2 out]
              n269 = Unbundle By Name(w224) -> ("Al Run"=w223:bool, "Prep Al"=w222:bool)
              n270 = call "flow_strings.vi"("string in"=w231, "is first in?"=TRUE, "use source?"=w225, "name"="Al", "run source?"=w223, "prep source?"=w222, "is prep?"=w226) -> ("string out"=w230:string, "is first out?"=w229:bool)
              n271 = property on="Status Out" class="Str"("Value"=w230) -> ()  [unwired: 2 in, 2 out]
              n272 = property on="first" class="Bool (strict)"("Value"=w229) -> ()  [unwired: 2 in, 2 out]
            }
            frame #2 {
              n273 = property on="main" class="Clust (strict)"() -> ("Value"=w234:T18)  [unwired: 2 in, 2 out]
              n274 = property on="Active" class="Bool (strict)"() -> ("Value"=w235:bool)  [unwired: 2 in, 2 out]
              n275 = property on="first" class="Bool (strict)"() -> ("Value"=w238:bool)  [unwired: 2 in, 2 out]
              n276 = property on="Status Out" class="Str"() -> ("Value"=w240:string)  [unwired: 2 in, 2 out]
              n277 = Unbundle By Name(w234) -> ("Run"=w233:bool, "Prep Ga"=w232:bool)
              n278 = call "flow_strings.vi"("string in"=w240, "is first in?"=w238, "use source?"=w235, "name"="Ga", "run source?"=w233, "prep source?"=w232, "is prep?"=w236) -> ("string out"=w241:string, "is first out?"=w237:bool)
              n279 = property on="Status Out" class="Str"("Value"=w241) -> ()  [unwired: 2 in, 2 out]
              n280 = property on="first" class="Bool (strict)"("Value"=w237) -> ()  [unwired: 2 in, 2 out]
            }
            frame #3 {
              n281 = property on="In bubbler Active" class="Bool (strict)"() -> ("Value"=w245:bool)  [unwired: 2 in, 2 out]
              n282 = property on="In main" class="Clust (strict)"() -> ("Value"=w244:T19)  [unwired: 2 in, 2 out]
              n283 = property on="first" class="Bool (strict)"() -> ("Value"=w249:bool)  [unwired: 2 in, 2 out]
              n284 = property on="Status Out" class="Str"() -> ("Value"=w251:string)  [unwired: 2 in, 2 out]
              n285 = Unbundle By Name(w244) -> ("In Run"=w243:bool, "Prep In"=w242:bool)
              n286 = call "flow_strings.vi"("string in"=w251, "is first in?"=w249, "use source?"=w245, "name"="In", "run source?"=w243, "prep source?"=w242, "is prep?"=w246) -> ("string out"=w248:string, "is first out?"=w247:bool)
              n287 = property on="Status Out" class="Str"("Value"=w248) -> ()  [unwired: 2 in, 2 out]
              n288 = property on="first" class="Bool (strict)"("Value"=w247) -> ()  [unwired: 2 in, 2 out]
            }
            frame #4 {
              n289 = property on="P gas Active" class="Bool (strict)"() -> ("Value"=w255:bool)  [unwired: 2 in, 2 out]
              n290 = property on="P gas main" class="Clust (strict)"() -> ("Value"=w254:T20)  [unwired: 2 in, 2 out]
              n291 = property on="first" class="Bool (strict)"() -> ("Value"=w258:bool)  [unwired: 2 in, 2 out]
              n292 = property on="Status Out" class="Str"() -> ("Value"=w260:string)  [unwired: 2 in, 2 out]
              n293 = Unbundle By Name(w254) -> ("PH3 Run"=w253:bool, "PH3 Prep"=w252:bool)
              n294 = call "flow_strings.vi"("string in"=w260, "is first in?"=w258, "use source?"=w255, "name"="PH3", "run source?"=w253, "prep source?"=w252, "is prep?"=w256) -> ("string out"=w259:string, "is first out?"=w257:bool)
              n295 = property on="Status Out" class="Str"("Value"=w259) -> ()  [unwired: 2 in, 2 out]
              n296 = property on="first" class="Bool (strict)"("Value"=w257) -> ()  [unwired: 2 in, 2 out]
            }
            frame #5 {
              n297 = property on="As gas Active" class="Bool (strict)"() -> ("Value"=w265:bool)  [unwired: 2 in, 2 out]
              n298 = property on="As gas main" class="Clust (strict)"() -> ("Value"=w264:T21)  [unwired: 2 in, 2 out]
              n299 = property on="first" class="Bool (strict)"() -> ("Value"=w268:bool)  [unwired: 2 in, 2 out]
              n300 = property on="Status Out" class="Str"() -> ("Value"=w270:string)  [unwired: 2 in, 2 out]
              n301 = Unbundle By Name(w264) -> ("AsH3 Run"=w263:bool, "AsH3 Prep"=w262:bool)
              n302 = call "flow_strings.vi"("string in"=w270, "is first in?"=w268, "use source?"=w265, "name"="AsH3", "run source?"=w263, "prep source?"=w262, "is prep?"=w266) -> ("string out"=w267:string, "is first out?"=w269:bool)
              n303 = property on="Status Out" class="Str"("Value"=w267) -> ()  [unwired: 2 in, 2 out]
              n304 = property on="first" class="Bool (strict)"("Value"=w269) -> ()  [unwired: 2 in, 2 out]
            }
            frame #6 {
              n305 = property on="P bubbler main" class="Clust (strict)"() -> ("Value"=w274:T22)  [unwired: 2 in, 2 out]
              n306 = property on="P bubbler Active" class="Bool (strict)"() -> ("Value"=w275:bool)  [unwired: 2 in, 2 out]
              n307 = Unbundle By Name(w274) -> ("P bubbler Run"=w273:bool, "P bubbler Prep"=w272:bool)
              n308 = property on="first" class="Bool (strict)"() -> ("Value"=w279:bool)  [unwired: 2 in, 2 out]
              n309 = property on="Status Out" class="Str"() -> ("Value"=w281:string)  [unwired: 2 in, 2 out]
              n310 = call "flow_strings.vi"("string in"=w281, "is first in?"=w279, "use source?"=w275, "name"="P liq", "run source?"=w273, "prep source?"=w272, "is prep?"=w276) -> ("string out"=w278:string, "is first out?"=w277:bool)
              n311 = property on="Status Out" class="Str"("Value"=w278) -> ()  [unwired: 2 in, 2 out]
              n312 = property on="first" class="Bool (strict)"("Value"=w277) -> ()  [unwired: 2 in, 2 out]
            }
            frame #7 {
              n313 = property on="main" class="Clust (strict)"() -> ("Value"=w284:T18)  [unwired: 2 in, 2 out]
              n314 = property on="Active" class="Bool (strict)"() -> ("Value"=w285:bool)  [unwired: 2 in, 2 out]
              n315 = property on="first" class="Bool (strict)"() -> ("Value"=w289:bool)  [unwired: 2 in, 2 out]
              n316 = property on="Status Out" class="Str"() -> ("Value"=w291:string)  [unwired: 2 in, 2 out]
              n317 = Unbundle By Name(w284) -> ("Run"=w283:bool, "Prep Ga"=w282:bool)
              n318 = call "flow_strings.vi"("string in"=w291, "is first in?"=w289, "use source?"=w285, "name"="Se", "run source?"=w283, "prep source?"=w282, "is prep?"=w286) -> ("string out"=w288:string, "is first out?"=w287:bool)
              n319 = property on="Status Out" class="Str"("Value"=w288) -> ()  [unwired: 2 in, 2 out]
              n320 = property on="first" class="Bool (strict)"("Value"=w287) -> ()  [unwired: 2 in, 2 out]
            }
          }
        }
        frame #3 {
          n321 = property on="prep_done" class="Bool (strict)"() -> ("Value"=w298:bool)  [unwired: 2 in, 2 out]
          n322 = property on="run started" class="Bool (strict)"() -> ("Value"=w297:bool)  [unwired: 2 in, 2 out]
          n323 = Not(x=w297) -> (.not. x?=w296:bool)
          n324 = And(x=w298, y=w296) -> (x .and. y?=w292:bool)
          n325 = case shown="True" w292 {
            selector: w292 -> [_ w300]
            tunnel: w295 -> [w299 w303]
            tunnel: [w299 w302] -> w294
            tunnel: w293 -> [_ w301]
            frame False {
            }
            frame True {
              n326 = stacked-sequence {
                tunnel: w301 -> [w305 _]
                tunnel: w303 -> [_ w315]
                tunnel: [_ w314] -> w302
                tunnel: w300 -> [w304 _]
                frame #0 {
                  n327 = case shown="False" w305 {
                    tunnel: w304 -> [w307 _]
                    frame False {
                      n328 = property on="In bubbler" class="Clust (strict)"() -> ("Value"=w311:T8)  [unwired: 2 in, 2 out]
                      n329 = property on="Ga bubbler" class="Clust (strict)"() -> ("Value"=w312:T16)  [unwired: 2 in, 2 out]
                      n330 = property on="Al bubbler" class="Clust (strict)"() -> ("Value"=w313:T11)  [unwired: 2 in, 2 out]
                      n331 = property on="Se bubbler" class="Clust (strict)"() -> ("Value"=w306:T16)  [unwired: 2 in, 2 out]
                      n332 = property on="P gas" class="Clust (strict)"() -> ("Value"=w310:T6)  [unwired: 2 in, 2 out]
                      n333 = property on="As gas" class="Clust (strict)"() -> ("Value"=w309:T4)  [unwired: 2 in, 2 out]
                      n334 = property on="P bubbler" class="Clust (strict)"() -> ("Value"=w308:T2)  [unwired: 2 in, 2 out]
                      n335 = call "Set_V_III.vi"("Se bubbler"=w306, "P bubbler"=w308, "As gas"=w309, "P gas"=w310, "Run Started"=w307, "In bubbler"=w311, "Ga bubbler"=w312, "Al bubbler"=w313) -> ()  [unwired: 4 in]
                    }
                    frame True {
                    }
                  }
                }
                frame #1 {
                  n336 = call "Set_Argument.vi"("Enable"=TRUE, "Argument"="run_started", "Argument List In"=w315) -> ("Argument List Out"=w314:string[])
                }
              }
            }
          }
        }
      }
    }
    frame "End" {
    }
    frame "Idle" {
    }
  }
  "Argument List Out" <- w10
